vi "Free.vi"(8 "error in (no error)":errorcluster caption="错误输入（无错误）", 11 "FIFO(DBL) 输入":refnum<class "FIFO(I16).lvclass"> caption="DNL_LabVIEW Object in") -> (0 "error out":errorcluster caption="错误输出")   [LabVIEW 2012, in "FIFO(I16).lvclass"]
uses:
  FIFO(I16).lvclass
  FIFO(I16).lvclass/FIFO(I16).ctl
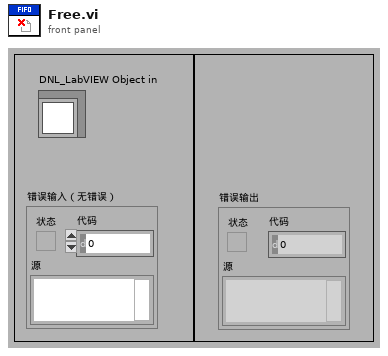
[diagram p1: front panel]
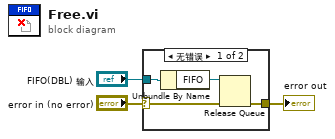
[diagram p0: block diagram]
diagram:
  n1 = case shown="无错误" "error in (no error)" {
    selector: "error in (no error)" -> [w5 w8]
    tunnel: [w4 w8] -> w2
    tunnel: "FIFO(DBL) 输入" -> [w7 _]
    frame No Error {
      n2 = Unbundle By Name(w7) -> ("FIFO"=w6:refnum<queue>)
      n3 = Release Queue(queue=w6, error in (no error)=w5) -> (error out=w4:errorcluster)  [unwired: 1 in, 2 out]
    }
    frame Error {
    }
  }
  "error out" <- w2
